vi "ResultJudge.vi"(8 "error in":errorcluster caption="错误输入", 9 "带卡？":bool, 11 "StrIn":string) -> (0 "error out":errorcluster caption="错误输出", 3 "StrOut":string)   [LabVIEW 2013]
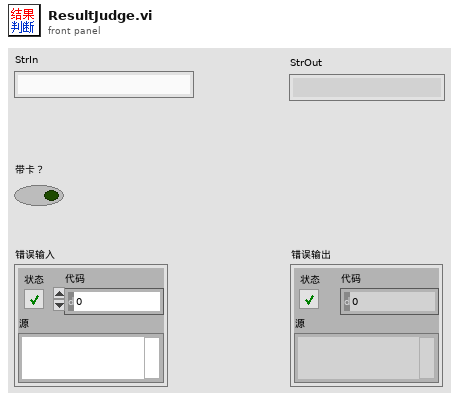
[diagram p1: front panel]
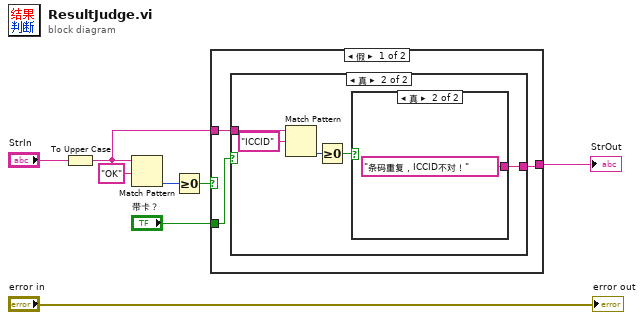
[diagram p0: block diagram]
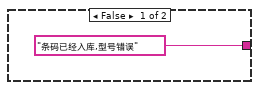
[diagram p2: hidden frame]
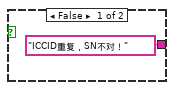
[diagram p3: hidden frame]
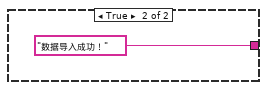
[diagram p4: hidden frame]
diagram:
  n1 = To Upper Case(1:"StrIn") -> (0:w3:string)
  n2 = Match Pattern(string=w3, regular expression="OK") -> (offset past match=w6:i32)  [unwired: 1 in, 3 out]
  n3 = Greater Or Equal To 0?(x=w6) -> (x >= 0?=w5:bool)
  n4 = case shown="假" w5 {
    tunnel: [w10 "数据导入成功！"] -> w4
    tunnel: w3 -> [w11 _]
    tunnel: "带卡？" -> [w9 _]
    frame False {
      n5 = case shown="真" w9 {
        tunnel: w11 -> [_ w17]
        tunnel: ["条码已经入库,型号错误" w13] -> w10
        frame False {
        }
        frame True {
          n6 = Match Pattern(string=w17, regular expression="ICCID" ("正则表达式")) -> (offset past match=w15:i32)  [unwired: 1 in, 3 out]
          n7 = Greater Or Equal To 0?(x=w15) -> (x >= 0?=w14:bool)
          n8 = case shown="真" w14 {
            tunnel: ["ICCID重复，SN不对！" "条码重复，ICCID不对！"] -> w13
            frame False {
            }
            frame True {
            }
          }
        }
      }
    }
    frame True {
    }
  }
  "StrOut" <- w4
  "error out" <- "error in"
